vi "pack DRAM data.vi"(8 "input valid?":bool, 9 "data to be packed":u32, 10 "DRAM Index in":T1, 11 "packer in":T2) -> (0 "output valid?":bool, 2 "DRAM Index out":T1, 3 "packer out":T2)   [LabVIEW 2015]
uses:
  DRAM data index.ctl
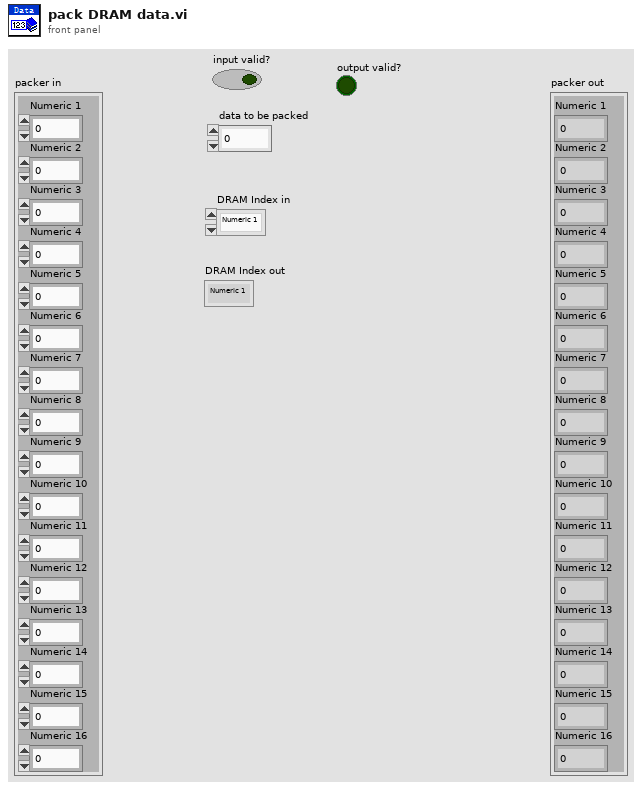
[diagram p1: front panel]
types:
  T1 = typedef "DRAM data index.ctl" = enum16{"Numeric 1", "Numeric 2", "Numeric 3", "Numeric 4", "Numeric 5", "Numeric 6", "Numeric 7", "Numeric 8", "Numeric 9", "Numeric 10", "Numeric 11", "Numeric 12", "Numeric 13", "Numeric 14", "Numeric 15", "Numeric 16"}
  T2 = cluster{"Numeric 1":u32, "Numeric 2":u32, "Numeric 3":u32, "Numeric 4":u32, "Numeric 5":u32, "Numeric 6":u32, "Numeric 7":u32, "Numeric 8":u32, "Numeric 9":u32, "Numeric 10":u32, "Numeric 11":u32, "Numeric 12":u32, "Numeric 13":u32, "Numeric 14":u32, "Numeric 15":u32, "Numeric 16":u32}
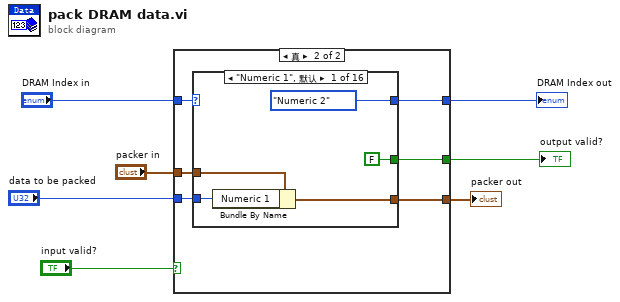
[diagram p0: block diagram]
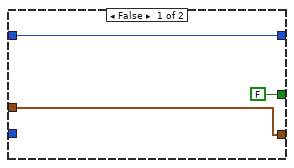
[diagram p2: hidden frame]
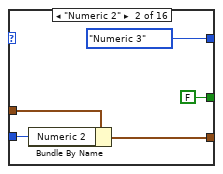
[diagram p3: hidden frame]
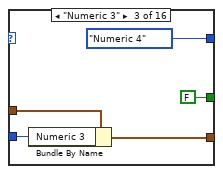
[diagram p4: hidden frame]
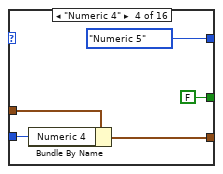
[diagram p5: hidden frame]
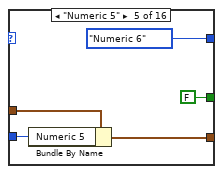
[diagram p6: hidden frame]
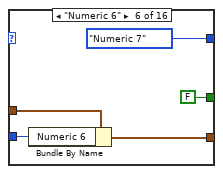
[diagram p7: hidden frame]
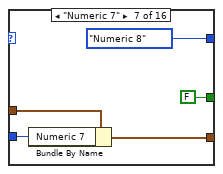
[diagram p8: hidden frame]
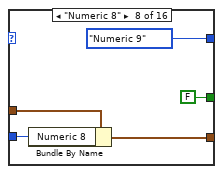
[diagram p9: hidden frame]
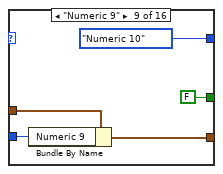
[diagram p10: hidden frame]
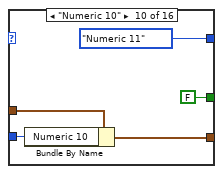
[diagram p11: hidden frame]
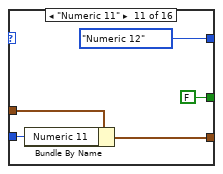
[diagram p12: hidden frame]
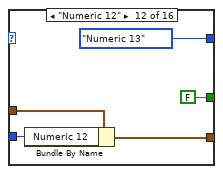
[diagram p13: hidden frame]
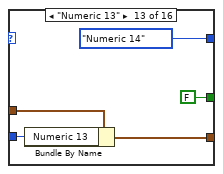
[diagram p14: hidden frame]
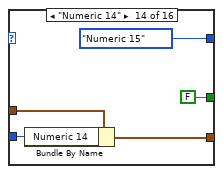
[diagram p15: hidden frame]
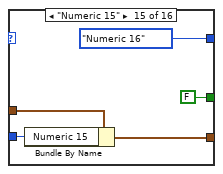
[diagram p16: hidden frame]
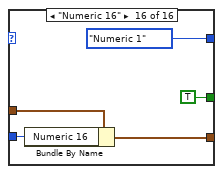
[diagram p17: hidden frame]
diagram:
  n1 = case shown="真" "input valid?" {
    tunnel: "DRAM Index in" -> [w8 w16]
    tunnel: "data to be packed" -> [_ w15]
    tunnel: [w8 w14] -> w1
    tunnel: "packer in" -> [w10 w13]
    tunnel: [w10 w12] -> w5
    tunnel: [FALSE w11] -> w4
    frame False {
    }
    frame True {
      n2 = case shown="\"Numeric 1\", 默认" w16 {
        tunnel: w13 -> [w20 w26 w31 w36 w41 w46 w51 w56 w61 w66 w71 w76 w81 w86 w91 w96]
        tunnel: [w19 w25 w30 w35 w40 w45 w50 w55 w60 w65 w70 w75 w80 w85 w90 w95] -> w12
        tunnel: [DRAM_data_index."Numeric 2" ("Galvo index in") DRAM_data_index."Numeric 3" ("Galvo index in") DRAM_data_index."Numeric 4" ("Galvo index in") DRAM_data_index."Numeric 5" ("Galvo index in") DRAM_data_index."Numeric 6" ("Galvo index in") DRAM_data_index."Numeric 7" ("Galvo index in") DRAM_data_index."Numeric 8" ("Galvo index in") DRAM_data_index."Numeric 9" ("Galvo index in") DRAM_data_index."Numeric 10" ("Galvo index in") DRAM_data_index."Numeric 11" ("Galvo index in") DRAM_data_index."Numeric 12" ("Galvo index in") DRAM_data_index."Numeric 13" ("Galvo index in") DRAM_data_index."Numeric 14" ("Galvo index in") DRAM_data_index."Numeric 15" ("Galvo index in") DRAM_data_index."Numeric 16" ("Galvo index in") DRAM_data_index."Numeric 1" ("Galvo index in")] -> w14
        tunnel: w15 -> [w21 w24 w29 w34 w39 w44 w49 w54 w59 w64 w69 w74 w79 w84 w89 w94]
        tunnel: [FALSE FALSE FALSE FALSE FALSE FALSE FALSE FALSE FALSE FALSE FALSE FALSE FALSE FALSE FALSE TRUE] -> w11
        frame "Numeric 1", Default {
          n3 = Bundle By Name(cluster=w20, "Numeric 1"=w21) -> (w19:T2)
        }
        frame "Numeric 2" {
          n4 = Bundle By Name(cluster=w26, "Numeric 2"=w24) -> (w25:T2)
        }
        frame "Numeric 3" {
          n5 = Bundle By Name(cluster=w31, "Numeric 3"=w29) -> (w30:T2)
        }
        frame "Numeric 4" {
          n6 = Bundle By Name(cluster=w36, "Numeric 4"=w34) -> (w35:T2)
        }
        frame "Numeric 5" {
          n7 = Bundle By Name(cluster=w41, "Numeric 5"=w39) -> (w40:T2)
        }
        frame "Numeric 6" {
          n8 = Bundle By Name(cluster=w46, "Numeric 6"=w44) -> (w45:T2)
        }
        frame "Numeric 7" {
          n9 = Bundle By Name(cluster=w51, "Numeric 7"=w49) -> (w50:T2)
        }
        frame "Numeric 8" {
          n10 = Bundle By Name(cluster=w56, "Numeric 8"=w54) -> (w55:T2)
        }
        frame "Numeric 9" {
          n11 = Bundle By Name(cluster=w61, "Numeric 9"=w59) -> (w60:T2)
        }
        frame "Numeric 10" {
          n12 = Bundle By Name(cluster=w66, "Numeric 10"=w64) -> (w65:T2)
        }
        frame "Numeric 11" {
          n13 = Bundle By Name(cluster=w71, "Numeric 11"=w69) -> (w70:T2)
        }
        frame "Numeric 12" {
          n14 = Bundle By Name(cluster=w76, "Numeric 12"=w74) -> (w75:T2)
        }
        frame "Numeric 13" {
          n15 = Bundle By Name(cluster=w81, "Numeric 13"=w79) -> (w80:T2)
        }
        frame "Numeric 14" {
          n16 = Bundle By Name(cluster=w86, "Numeric 14"=w84) -> (w85:T2)
        }
        frame "Numeric 15" {
          n17 = Bundle By Name(cluster=w91, "Numeric 15"=w89) -> (w90:T2)
        }
        frame "Numeric 16" {
          n18 = Bundle By Name(cluster=w96, "Numeric 16"=w94) -> (w95:T2)
        }
      }
    }
  }
  "packer out" <- w5
  "output valid?" <- w4
  "DRAM Index out" <- w1
